vi "params_tanslation.vi"(0 "params":T1(array[cluster])) -> (1 "output hex string":string, 2 "tablica charow (u8)":u8[](array[numeric]))   [LabVIEW 2012]
panel:
  out "przetworzona tablica charow (typu string)":string[](array[string])
  out "ilosc charow":u64
  out "ilosc bitow":i32
  out "suma bitow":u64
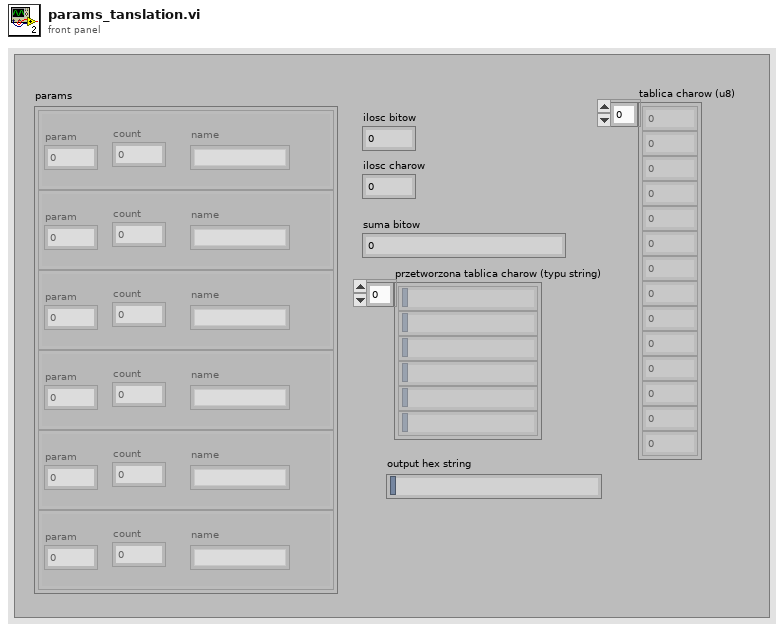
[diagram p1: front panel]
types:
  T1 = cluster{"param":u64, "count":u8, "name":string}[]
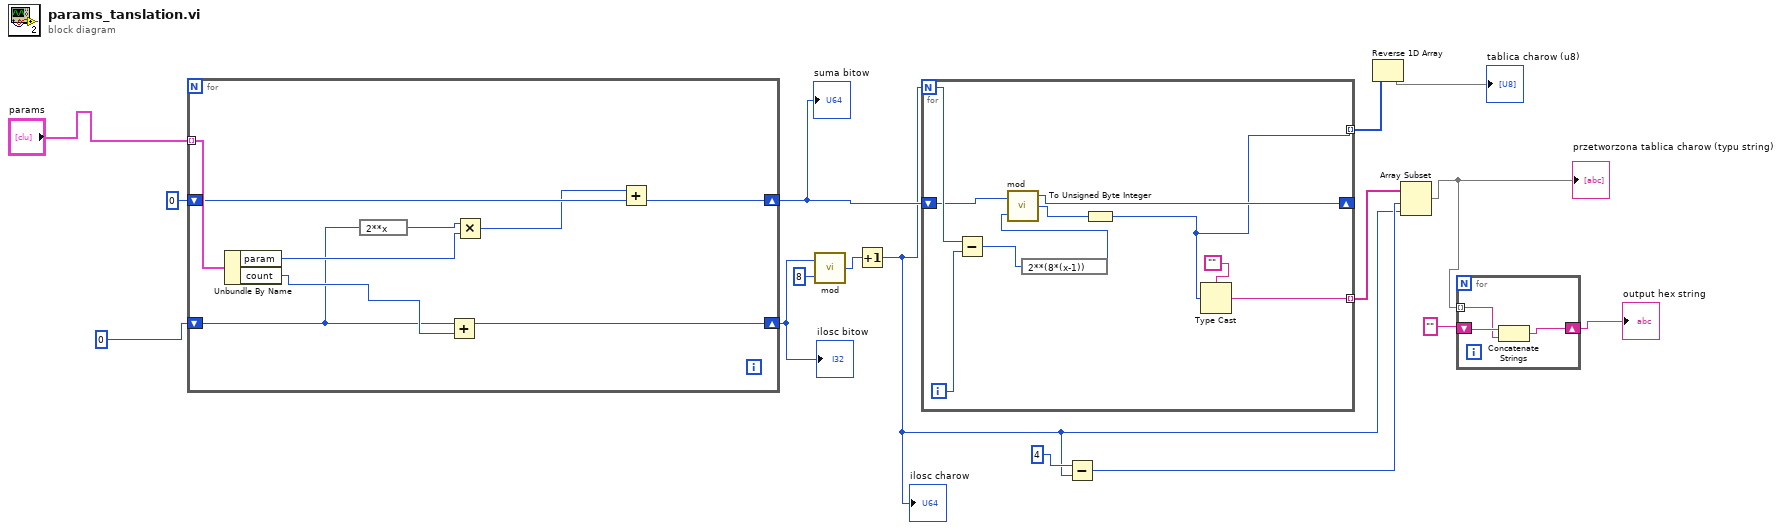
[diagram p0: block diagram]
diagram:
  n1 = for {
    tunnel: "params" -> [w25] mode=indexing
    shift-right: [w24] -> w13
    shift-left: 0 ("index") -> [w20]
    shift-right: [w18] -> w10
    shift-left: u64 0 -> [w19]
    n2 = Unbundle By Name(w25) -> ("param"=w21:u64, "count"=w23:u8)
    n3 = expression code="2**x"(w20) -> (w22:i32)
    n4 = Add(x=w20, y=w23) -> (x+y=w24:i32)
    n5 = Multiply(x=w22, y=w21) -> (x*y=w17:u64)
    n6 = Add(x=w17, y=w19) -> (x+y=w18:u64)
  }
  "suma bitow" <- w10
  "ilosc bitow" <- w13
  n7 = call "mod.vi"("number"=w13, "dzielnik"=u64 8) -> ("czesc calkowita"=w11:u64)  [unwired: 2 out]
  n8 = Increment(x=w11) -> (x+1=w3:u64)
  "ilosc charow" <- w3
  n9 = for {
    N: w3 -> [w35]
    shift-right: [w32] -> _
    shift-left: w10 -> [w28]
    tunnel: [w29] -> w9 mode=indexing
    tunnel: [w26] -> w2 mode=indexing
    i -> [w34]
    n10 = Subtract(x=w35, y=w34) -> (x-y=w27:u64)
    n11 = expression code="2**(8*(x-1))"(w27) -> (w33:u64)
    n12 = call "mod.vi"("number"=w28, "dzielnik"=w33) -> ("reszta"=w32:u64, "czesc calkowita"=w31:u64)  [unwired: 1 out]
    n13 = To Unsigned Byte Integer(number=w31) -> (unsigned 8bit integer=w26:u8)
    n14 = Type Cast(type="", x=w26) -> (*(type *) &x=w29:string)
  }
  n15 = Subtract(x=u64 4 ("y"), y=w3) -> (x-y=w8:u64)
  n16 = Reverse 1D Array(array=w2) -> (reversed array=→"tablica charow (u8)":u8[])
  n17 = Array Subset(array=w9, index=w8, length=w3) -> (w6:string[])
  "przetworzona tablica charow (typu string)" <- w6
  n18 = for {
    tunnel: w6 -> [w37] mode=indexing
    shift-right: [w36] -> w4
    shift-left: "" ("output hex string") -> [w38]
    n19 = Concatenate Strings(w38, w37) -> (w36:string)
  }
  "output hex string" <- w4
